vi "CAN Excel Read.vi"(11 "DBC Define":path=path "C:/Users/26832/Desktop/SHQC/SHQC.xlsx") -> ()   [LabVIEW 2020]
uses:
  <vilib>/Utility/file.llb/Write Delimited Spreadsheet (string).vi
panel:
  in  "簇":T1
  out "CAN":string[][](table)
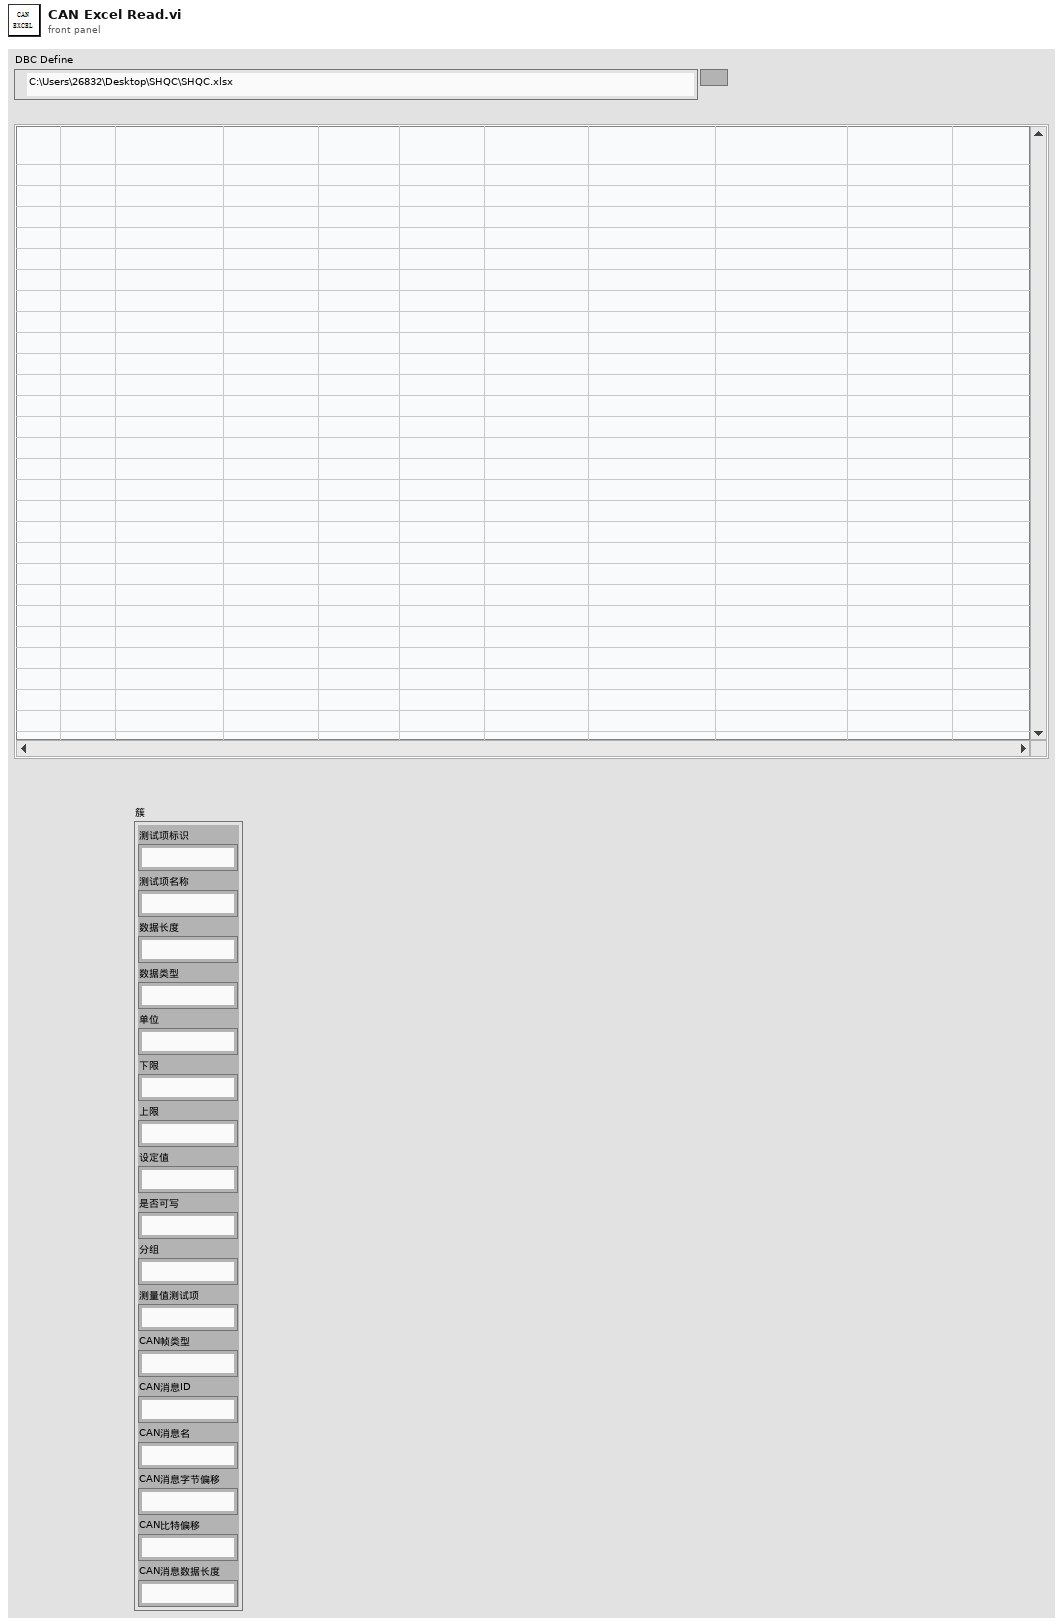
[diagram p1: front panel]
types:
  T1 = cluster{"测试项标识":string, "测试项名称":string, "数据长度":string, "数据类型":string, "单位":string, "下限":string, "上限":string, "设定值":string, "是否可写":string, "分组":string, "测量值测试项":string, "CAN帧类型":string, "CAN消息ID":string, "CAN消息名":string, "CAN消息字节偏移":string, "CAN比特偏移":string, "CAN消息数据长度":string}
  T2 = cluster{"测试项标识":string, "测试项名称":string, "数据类型":string, "长度(bit)":string, "测试项类型":string, "单位":string, "下限":string, "上限":string, "是否可写":string, "转换系数":string, "转换偏量":string, "分组":string, "开始位置":string}
  T3 = cluster{"Start":i32, "Type":string, "W?":string, "Message ID":i32}
  T4 = cluster{"Message ID":string, "CANType":string, "MessageName":string, "MessageSize":string, "Transmitter":string, "SendType":string, "CycleTime(ms)":string}
  T5 = cluster{"Comment":string, "SignalName":string, "MultiplexorType":string, "MultiplexValue":string, "LSB(StartBit)":string, "SignalSize":string, "ByteOrder":string, "ValueType":string, "Factor":string, "Offset":string, "Min":string, "Max":string, "InitialValue":string, "InvalidHex":string, "Unit":string, "Meaning":string}
  T6 = cluster{"All[0]":string, "All[1]":string, "All[2]":string, "All[3]":string, "All[4]":string, "All[5]":string, "All[6]":string, "All[7]":string, "All[8]":string, "All[9]":string, "All[10]":string, "All[11]":string, "All[12]":string}
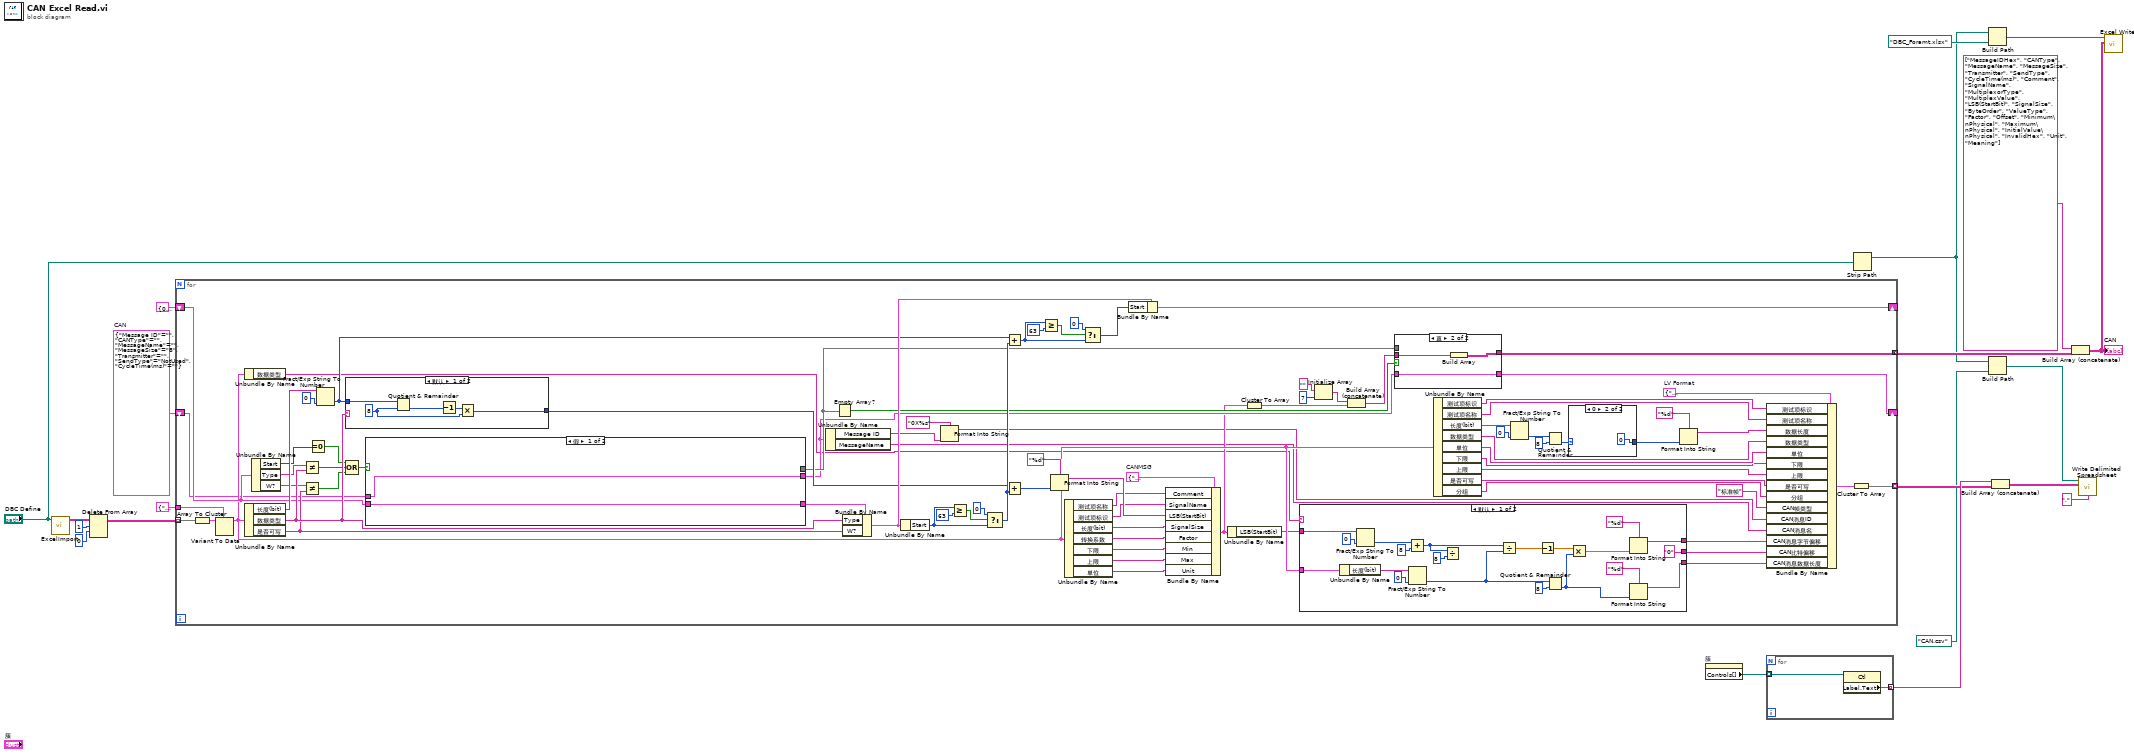
[diagram p0: block diagram]
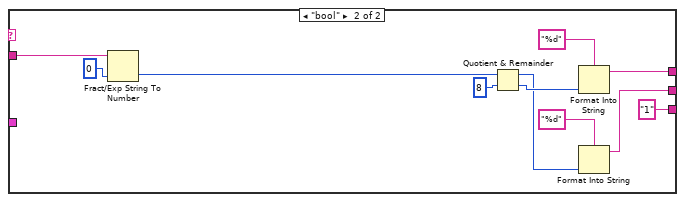
[diagram p2: hidden frame]
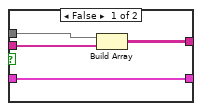
[diagram p4: hidden frame]
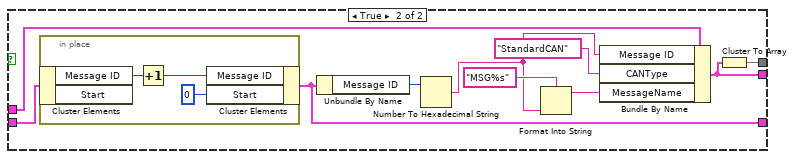
[diagram p5: hidden frame]
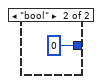
[diagram p6: hidden frame]
diagram:
  w12 = T4 {"Message ID"="", "CANType"="", "MessageName"="", "MessageSize"="8", "Transmitter"="", "SendType"="NotUsed", "CycleTime(ms)"=""}  # CAN
  n1 = call "ExcelImport.vi"("路径"="DBC Define") -> ("All"=w16:string[][])  [unwired: 7 in, 3 out]
  n2 = Delete From Array(array=w16, length=1 ("长度"), index (row)=0 ("索引 (行)")) -> (array with subset deleted=w19:string[][])  [unwired: 1 in, 1 out]
  n3 = for {
    tunnel: w19 -> [w104] mode=indexing
    tunnel: T2 {"测试项标识"="", "测试项名称"="", "数据类型"="", "长度(bit)"="", "测试项类型"="", "单位"="", "下限"="", "上限"="", "是否可写"="", "转换系数"="", "转换偏量"="", "分组"="", "开始位置"=""} -> [w102]
    shift-right: [w83] -> _
    shift-left: T3 {"Start"=0, "Type"="", "W?"="", "Message ID"=47} -> [w72]
    tunnel: [w82] -> w10 mode=concatenating
    shift-right: [w62] -> _
    shift-left: w12 -> [w58]
    tunnel: [w59] -> w6 mode=indexing
    w22 = T1 {"测试项标识"="", "测试项名称"="", "数据长度"="", "数据类型"="", "单位"="", "下限"="", "上限"="", "设定值"="", "是否可写"="", "分组"="", "测量值测试项"="", "CAN帧类型"="", "CAN消息ID"="", "CAN消息名"="", "CAN消息字节偏移"="", "CAN比特偏移"="", "CAN消息数据长度"=""}  # LV Format
    w23 = T5 {"Comment"="", "SignalName"="", "MultiplexorType"="Normal Signal", "MultiplexValue"="", "LSB(StartBit)"="", "SignalSize"="", "ByteOrder"="Motorola", "ValueType"="Unsigned", "Factor"="1", "Offset"="0", "Min"="", "Max"="", "InitialValue"="", "InvalidHex"="", "Unit"="", "Meaning"=""}  # CANMSG
    n4 = Array To Cluster(array=w104) -> (cluster=w103:T6)
    n5 = Variant To Data(type=w102, Variant=w103) -> (data=w63:T2)  [unwired: 1 in, 1 out]
    n6 = Unbundle By Name(w63) -> ("数据类型"=w35:string)
    n7 = Unbundle By Name(w63) -> ("长度(bit)"=w101:string, "数据类型"=w95:string, "是否可写"=w93:string)
    n8 = Unbundle By Name(w72) -> ("Start"=w70:i32, "Type"=w96:string, "W?"=w94:string)
    n9 = Not Equal?(x=w96, y=w95) -> (x != y?=w92:bool)
    n10 = Not Equal?(x=w94, y=w93) -> (x != y?=w91:bool)
    n11 = Equal To 0?(x=w70) -> (x = 0?=w69:bool)
    n12 = Fract/Exp String To Number(string=w101, default (0 dbl)=u32 0 ("默认(0 DBL)")) -> (number=w73:u32)  [unwired: 2 in, 1 out]
    n13 = case shown="默认" w95 {
      tunnel: w73 -> [w164 _]
      tunnel: [w160 u32 0] -> w87
      frame Default {
        w161 = u32 8 ("y")
        n14 = Quotient & Remainder(x=w164, y=w161) -> (floor(x/y)=w163:u32)  [unwired: 1 out]
        n15 = Decrement(x=w163) -> (x-1=w162:u32)
        n16 = Multiply(x=w162, y=w161) -> (x*y=w160:u32)
      }
      frame "bool" {
      }
    }
    n17 = Compound Arithmetic op=OR ("复合运算")(w69, w92, w91) -> (w85:bool)
    n18 = case shown="假" w85 {
      tunnel: w72 -> [w146 w156]
      tunnel: [w146 w153] -> w84
      tunnel: w58 -> [w145 w155]
      tunnel: [_ w154] -> w76
      tunnel: [w145 w152] -> w61
      frame False {
      }
      frame True {
        n19 = in-place {
          n20 = in-place-cluster #1(w156) -> ("Message ID"=w159:i32)  [unwired: 1 out]
          n21 = Increment(x=w159) -> (x+1=w158:i32)
          n22 = in-place-cluster #1("Message ID"=w158, "Start"=0) -> (w153:T3)
        }
        n23 = Unbundle By Name(w153) -> ("Message ID"=w151:i32)
        n24 = Number To Hexadecimal String(2:w151) -> (0:w148:string)  [unwired: 1 in]
        n25 = Format Into String(format string="MSG%s" ("格式字符串"), w148) -> (resulting string=w147:string)  [unwired: 2 in, 1 out]
        n26 = Bundle By Name(cluster=w155, "Message ID"=w148, "CANType"="StandardCAN", "MessageName"=w147) -> (w152:T4)
        n27 = Cluster To Array(cluster=w152) -> (array=w154:string[])
      }
    }
    n28 = Unbundle By Name(w61) -> ("Message ID"=w38:string, "MessageName"=w36:string)
    n29 = Empty Array?(array=w76) -> (empty?=w75:bool)
    n30 = Bundle By Name(cluster=w84, "Type"=w95, "W?"=w93) -> (w90:T3)
    n31 = Unbundle By Name(w90) -> ("Start"=w89:i32)
    n32 = Format Into String(format string="0X%s" ("格式字符串"), w38) -> (resulting string=w37:string)  [unwired: 2 in, 1 out]
    n33 = Greater Or Equal?(x=w89, y=u32 63) -> (x >= y?=w71:bool)
    n34 = Select(t=u32 0 ("y"), s=w71, f=w89) -> (s? t:f=w88:u32)
    n35 = Add(x=w73, y=w88) -> (x+y=w65:u32)
    n36 = Add(x=w87, y=w88) -> (x+y=w86:u32)
    n37 = Greater Or Equal?(x=w65, y=u32 63) -> (x >= y?=w68:bool)
    n38 = Format Into String(format string="%d" ("格式字符串"), w86) -> (resulting string=w74:string)  [unwired: 2 in, 1 out]
    n39 = Unbundle By Name(w63) -> ("测试项名称"=w30:string, "测试项标识"=w25:string, "长度(bit)"=w29:string, "转换系数"=w28:string, "下限"=w27:string, "上限"=w26:string, "单位"=w24:string)
    n40 = Select(t=u32 0 ("y"), s=w68, f=w65) -> (s? t:f=w64:u32)
    n41 = Bundle By Name(cluster=w90, "Start"=w64) -> (w83:T3)
    n42 = Bundle By Name(cluster=w23, "Comment"=w30, "SignalName"=w25, "LSB(StartBit)"=w74, "SignalSize"=w29, "Factor"=w28, "Min"=w27, "Max"=w26, "Unit"=w24) -> (w57:T5)
    n43 = Unbundle By Name(w57) -> ("LSB(StartBit)"=w32:string)
    n44 = Cluster To Array(cluster=w57) -> (array=w78:string[])
    n45 = case shown="默认" w35 {
      tunnel: w32 -> [w116 w132]
      tunnel: [w114 w129] -> w34
      tunnel: ["0" w126] -> w33
      tunnel: [w119 "1"] -> w31
      tunnel: w63 -> [w124 _]
      frame Default {
        n46 = Unbundle By Name(w124) -> ("长度(bit)"=w121:string)
        n47 = Fract/Exp String To Number(string=w116, default (0 dbl)=u32 0 ("偏移量")) -> (number=w113:u32)  [unwired: 2 in, 1 out]
        n48 = Add(x=w113, y=u32 8) -> (x+y=w109:u32)
        n49 = Fract/Exp String To Number(string=w121, default (0 dbl)=u32 0 ("偏移量")) -> (number=w111:u32)  [unwired: 2 in, 1 out]
        n50 = Divide(x=w109, y=u32 8) -> ()  [unwired: 1 out]
        n51 = Divide(x=w109, y=w111) -> (x/y=w110:dbl)
        n52 = Decrement(x=w110) -> (x-1=w107:dbl)
        n53 = Quotient & Remainder(x=w111, y=u32 8) -> (floor(x/y)=w106:u32)  [unwired: 1 out]
        n54 = Multiply(x=w107, y=w106) -> (x*y=w105:dbl)
        n55 = Format Into String(format string="%d" ("格式字符串"), w105) -> (resulting string=w114:string)  [unwired: 2 in, 1 out]
        n56 = Format Into String(format string="%d" ("格式字符串"), w106) -> (resulting string=w119:string)  [unwired: 2 in, 1 out]
      }
      frame "bool" {
        n57 = Fract/Exp String To Number(string=w132, default (0 dbl)=u32 0 ("偏移量")) -> (number=w133:u32)  [unwired: 2 in, 1 out]
        n58 = Quotient & Remainder(x=w133, y=u32 8) -> (x-y*floor(x/y)=w127:u32, floor(x/y)=w130:u32)
        n59 = Format Into String(format string="%d" ("格式字符串"), w130) -> (resulting string=w129:string)  [unwired: 2 in, 1 out]
        n60 = Format Into String(format string="%d" ("格式字符串"), w127) -> (resulting string=w126:string)  [unwired: 2 in, 1 out]
      }
    }
    n61 = Initialize Array("", 7 ("维数大小")) -> (w79:string[])
    n62 = Build Array (concatenate)(w79, w78) -> (w77:string[])
    n63 = case shown="真" w75 {
      tunnel: [w141 w143] -> w82
      tunnel: w77 -> [w140 w144]
      tunnel: w76 -> [w139 _]
      tunnel: [w138 w142] -> w62
      tunnel: w61 -> [w138 w142]
      frame False {
        n64 = Build Array(w139, w140) -> (w141:string[][])
      }
      frame True {
        n65 = Build Array(w144) -> (w143:string[][])
      }
    }
    n66 = Unbundle By Name(w63) -> ("测试项标识"=w56:string, "测试项名称"=w55:string, "长度(bit)"=w54:string, "数据类型"=w46:string, "单位"=w45:string, "下限"=w44:string, "上限"=w43:string, "是否可写"=w42:string, "分组"=w41:string)
    n67 = Fract/Exp String To Number(string=w54, default (0 dbl)=u32 0 ("偏移量")) -> (number=w53:u32)  [unwired: 2 in, 1 out]
    n68 = Quotient & Remainder(x=w53, y=u32 8) -> (floor(x/y)=w50:u32)  [unwired: 1 out]
    n69 = case shown="0" w50 {
      selector: w50 -> [w136 _]
      tunnel: [w136 0] -> w48
      frame Default {
      }
      frame 0 {
      }
    }
    n70 = Format Into String(format string="%d" ("格式字符串"), w48) -> (resulting string=w47:string)  [unwired: 2 in, 1 out]
    n71 = Bundle By Name(cluster=w22, "测试项标识"=w56, "测试项名称"=w55, "数据长度"=w47, "数据类型"=w46, "单位"=w45, "下限"=w44, "上限"=w43, "是否可写"=w42, "分组"=w41, "CAN帧类型"="标准帧", "CAN消息ID"=w37, "CAN消息名"=w36, "CAN消息字节偏移"=w34, "CAN比特偏移"=w33, "CAN消息数据长度"=w31) -> (w60:T1)
    n72 = Cluster To Array(cluster=w60) -> (array=w59:string[])
  }
  n73 = property on="簇" class="Clust (严格)"() -> ("Controls[]"=w18:refnum<vi>[])  [unwired: 2 in, 2 out]
  n74 = for {
    tunnel: w18 -> [w167] mode=indexing
    tunnel: [w166] -> w15 mode=indexing
    n75 = property class="Ctl"(reference=w167) -> ("Label.Text"=w166:string)  [unwired: 1 in, 2 out]
  }
  n76 = Strip Path(path="DBC Define") -> (stripped path=w5:path)  [unwired: 1 out]
  n77 = Build Path(base path=w5, name or relative path=path "DBC_Foramt.xlsx" ("名称或相对路径")) -> (appended path=w7:path)
  n78 = Build Path(base path=w5, name or relative path=path "CAN.csv" ("名称或相对路径")) -> (appended path=w3:path)
  n79 = Build Array (concatenate)(w15, w6) -> (w2:string[][])
  n80 = Build Array (concatenate)(string[] ["MessageIDHex", "CANType", "MessageName", "MessageSize", "Transmitter", "SendType", "CycleTime(ms)", "Comment", "SignalName", "MultiplexorType", "MultiplexValue", "LSB(StartBit)", "SignalSize", "ByteOrder", "ValueType", "Factor", "Offset", "Minimum\nPhysical", "Maximum\nPhysical", "InitialValue\nPhysical", "InvalidHex", "Unit", "Meaning"] ("string array"), w10) -> (w9:string[][])
  "CAN" <- w9
  n81 = call-poly <vilib>:"Write Delimited Spreadsheet.vi"("file path (dialog if empty)"=w3, "2D data"=w2, "delimiter (\\t)"="," ("delimiter (\\t)")) -> ()  [unwired: 11 in, 2 out]
  n82 = call "Excel Write.vi"("Write"=w9, "Path"=w7) -> ()  [unwired: 9 in, 1 out]
